vi "Serialize.vi"   [LabVIEW 2020, in "NI_SFTP.lvlib" / "Low Level Connection.lvclass"]
uses:
  <vilib>/net/SFTP/Low Level Connection/Low Level Connection.lvclass
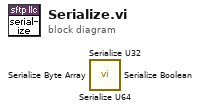
[diagram p0: block diagram]
diagram:
  n1 = call <vilib>:"Serialize U64.vi"() -> ()  [unwired: 3 in, 1 out]
  n2 = call <vilib>:"Serialize U32.vi"() -> ()  [unwired: 3 in, 1 out]
  n3 = call <vilib>:"Serialize Byte Array.vi"() -> ()  [unwired: 3 in, 1 out]
  n4 = call <vilib>:"Serialize Boolean.vi"() -> ()  [unwired: 3 in, 1 out]
